vi "Set Channel Outputs.vi"(7 "Channel Select (1)":u8=1 min=1 max=3, 8 "OVP":dbl, 9 "Amps":dbl, 10 "Volts":dbl, 11 "VISA session":refnum<visa-resource-name>) -> (0 "error out":errorcluster)   [LabVIEW 2010]
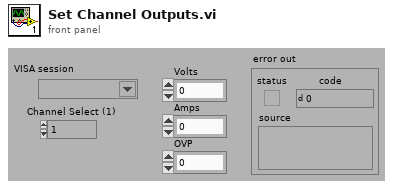
[diagram p1: front panel]
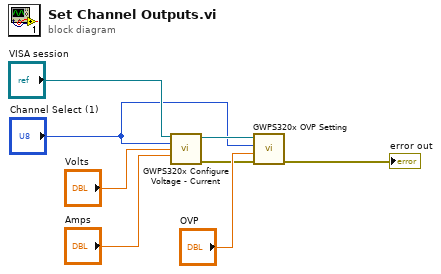
[diagram p0: block diagram]
diagram:
  n1 = call <instrlib>:"GWPS320x Configure Voltage - Current.vi"("VISA session"="VISA session", "Channel Select (1)"="Channel Select (1)", "Output Voltage (V) (0.0)"="Volts", "Output Current (A) (0.0)"="Amps") -> ("dup VISA session"=w5:refnum<visa-resource-name>, "error out"=w2:errorcluster)  [unwired: 10 in]
  n2 = call <instrlib>:"GWPS320x OVP Setting.vi"("error in (no error)"=w2, "OVP(V) (0.000)"="OVP", "Channel Select (1)"="Channel Select (1)", "VISA session"=w5) -> ("error out"=→"error out":errorcluster)  [unwired: 6 in, 1 out]
